vi "Release event log queue.vi"(8 "error in (no error)":errorcluster) -> (0 "error out":errorcluster, 3 "remaining elements":T1[](array[typedef]))   [LabVIEW 2020]
uses:
  Event log.ctl
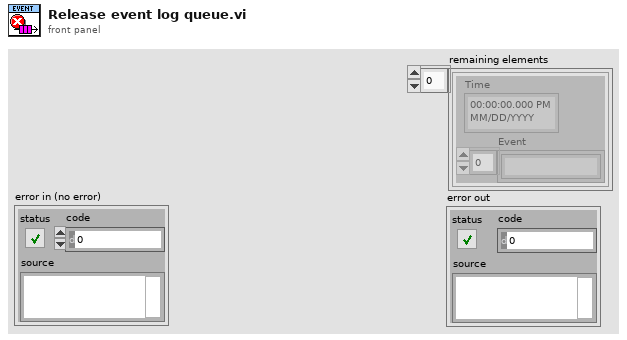
[diagram p1: front panel]
types:
  T1 = typedef "Event log.ctl" = cluster{"Time":timestamp, "Event":string[]}
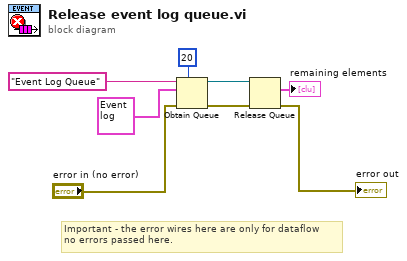
[diagram p0: block diagram]
diagram:
  # "Important - the error wires here are only for dataflow\nno errors passed here."
  n1 = Obtain Queue(max queue size (-1, unlimited)=20, name (unnamed)="Event Log Queue", element data type=T1 {"Time"=timestamp(0 s since 1904-01-01), "Event"=[]}, error in (no error)="error in (no error)") -> (queue out=w4:refnum<queue>, error out=w5:errorcluster)  [unwired: 1 in, 1 out]
  n2 = Release Queue(queue=w4, error in (no error)=w5) -> (remaining elements=→"remaining elements":T1[], error out=→"error out":errorcluster)  [unwired: 1 in, 1 out]
